vi "gl_User Events.vi"() -> ()   [LabVIEW 2020]
uses:
  Typedefs/Top level VI states.ctl
panel:
  out "User Events":T1
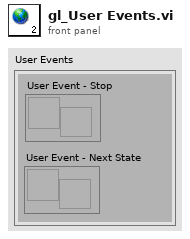
[diagram p1: front panel]
types:
  T1 = cluster{"User Event - Stop":refnum<user-event>, "User Event - Next State":refnum<user-event>}
diagram:
